vi "Configure Alarm Basic.vi"(0 "VISA resource name":refnum<visa-resource-name>, 1 "Individual Alarm ACK (0: Not Change)":u16(ring) items=["Not Change", "Disable", "Enable"], 5 "Rate Of Change Decrease (1)":i32=1 min=1 max=32, 7 "Rate Of Change Increase (1)":i32=1 min=1 max=32, 9 "Enable Holding Alarm Indicator (Disable)":bool, 11 "error in (no error)":errorcluster) -> (4 "VISA resource name out":refnum<visa-resource-name>, 15 "error out":errorcluster)   [LabVIEW 2020, in "Yokogawa GX Series.lvlib"]
doc: "Sets the alarm basic.\n\nCommands: SAlmLimit, SAlmSts"
uses:
  <instrlib>/Yokogawa GX Series/Yokogawa GX Series.lvlib
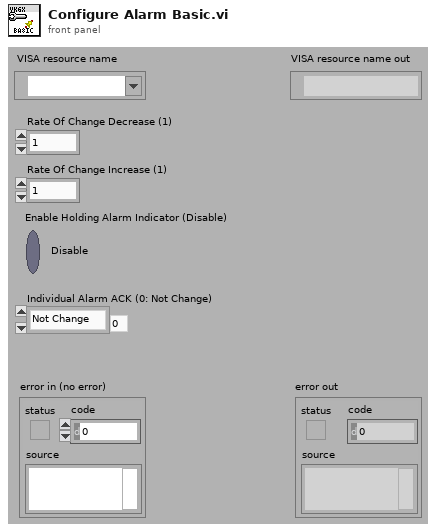
[diagram p1: front panel]
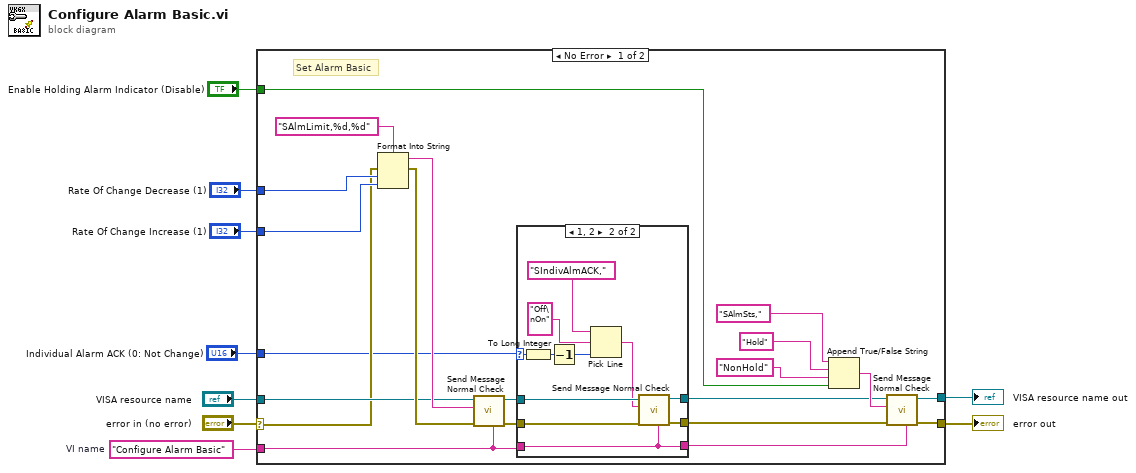
[diagram p0: block diagram]
diagram:
  w9 = "Configure Alarm Basic"  # VI name
  n1 = case shown="No Error" "error in (no error)" {
    selector: "error in (no error)" -> [w21 w45]
    tunnel: w9 -> [w11 _]
    tunnel: [w16 w46] -> w8
    tunnel: [w15 w45] -> w7
    tunnel: "Rate Of Change Decrease (1)" -> [w29 _]
    tunnel: "Rate Of Change Increase (1)" -> [w28 _]
    tunnel: "VISA resource name" -> [w25 w46]
    tunnel: "Individual Alarm ACK (0: Not Change)" -> [w19 _]
    tunnel: "Enable Holding Alarm Indicator (Disable)" -> [w12 _]
    frame No Error {
      # "Set Alarm Basic"
      n2 = Format Into String(format string="SAlmLimit,%d,%d", error in=w21, w29, w28) -> (resulting string=w26:string, error out=w27:errorcluster)  [unwired: 1 in]
      n3 = call <instrlib>:"Send Message Normal Check.vi"("Source (\"\")"=w11, "error in (no error)"=w27, "Send Message (\"\")"=w26, "VISA resource name"=w25) -> ("error out"=w17:errorcluster, "VISA resource name out"=w18:refnum<visa-resource-name>)  [unwired: 2 in, 4 out]
      n4 = case shown="1, 2" w19 {
        selector: w19 -> [_ w35]
        tunnel: w18 -> [w33 w44]
        tunnel: w17 -> [w32 w43]
        tunnel: [w33 w42] -> w14
        tunnel: [w32 w41] -> w13
        tunnel: w11 -> [w31 w34]
        tunnel: [w31 w34] -> w10
        frame 0, Default {
        }
        frame 1, 2 {
          n5 = To Long Integer(number=w35) -> (32bit integer=w36:i32)
          n6 = Decrement(x=w36) -> (x-1=w38:i32)
          n7 = Pick Line(string ("")="SIndivAlmACK,", multi-line string="Off\nOn", line index=w38) -> (output string=w37:string)
          n8 = call <instrlib>:"Send Message Normal Check.vi"("Source (\"\")"=w34, "error in (no error)"=w43, "Send Message (\"\")"=w37, "VISA resource name"=w44) -> ("error out"=w41:errorcluster, "VISA resource name out"=w42:refnum<visa-resource-name>)  [unwired: 2 in, 4 out]
        }
      }
      n9 = Append True/False String(1:w12, 2:"NonHold", 3:"Hold", 4:"SAlmSts,") -> (0:w20:string)
      n10 = call <instrlib>:"Send Message Normal Check.vi"("Source (\"\")"=w10, "error in (no error)"=w13, "Send Message (\"\")"=w20, "VISA resource name"=w14) -> ("error out"=w15:errorcluster, "VISA resource name out"=w16:refnum<visa-resource-name>)  [unwired: 2 in, 4 out]
    }
    frame Error {
    }
  }
  "error out" <- w7
  "VISA resource name out" <- w8
